vi "Check config.vi"(3 "error in (no error)":errorcluster, 4 "input cluster":T1 {"MaxLambdaCurrent [A]" format="%.2f"; "LambdaRates [A/min]" format="%.2f"; "MaxNormalCurrent [A]" format="%.2f"; "StabilitySetting [%]" format="%.2f"; "FieldCurrentRatio [T/A]" format="%.2f"; "SwitchWaitTime [s]" format="%.2f"; "SwitchHtrCurrent [mA]" format="%.2f"; "TrainRates [A/min]" format="%.2f"; "NormalRates [A/min]" format="%.2f"; "Breakpts [A]" format="%.2f"}, 5 "VISA session":refnum<visa-resource-name>="GPIB0::22::INSTR") -> (0 "error out":errorcluster, 1 "output cluster":T1 {"MaxLambdaCurrent [A]" format="%.2f"; "LambdaRates [A/min]" format="%.2f"; "MaxNormalCurrent [A]" format="%.2f"; "StabilitySetting [%]" format="%.2f"; "FieldCurrentRatio [T/A]" format="%.2f"; "SwitchWaitTime [s]" format="%.2f"; "SwitchHtrCurrent [mA]" format="%.2f"; "TrainRates [A/min]" format="%.2f"; "NormalRates [A/min]" format="%.2f"; "Breakpts [A]" format="%.2f"}, 2 "VISA session dup":refnum<visa-resource-name>)   [LabVIEW 2019]
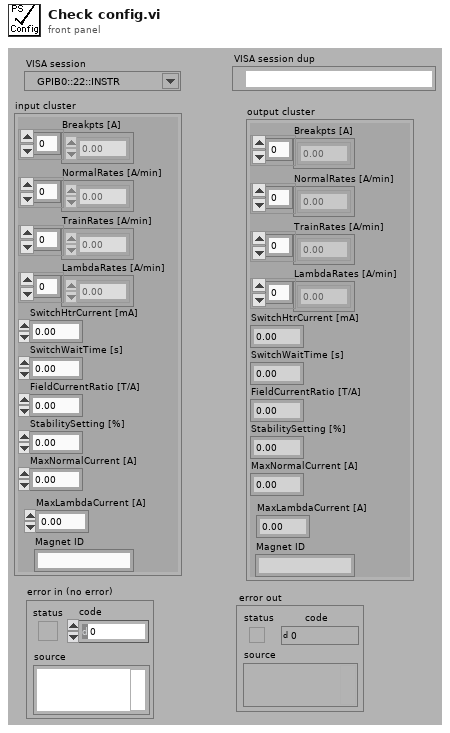
[diagram p1: front panel]
types:
  T1 = cluster{"Breakpts [A]":dbl[], "NormalRates [A/min]":dbl[], "TrainRates [A/min]":dbl[], "SwitchHtrCurrent [mA]":dbl, "SwitchWaitTime [s]":dbl, "FieldCurrentRatio [T/A]":dbl, "StabilitySetting [%]":dbl, "MaxNormalCurrent [A]":dbl, "Magnet ID":string, "LambdaRates [A/min]":dbl[], "MaxLambdaCurrent [A]":dbl}
  T2 = enum16{"SwitchHtrCurrent", "SwitchWaitTime", "FieldCurrentRatio", "StabilitySetting", "MaxNormalCurrent", "MaxLambdaCurrent"}
  T3 = enum16{"Normal", "Train", "Lambda", "Train & Lambda"}
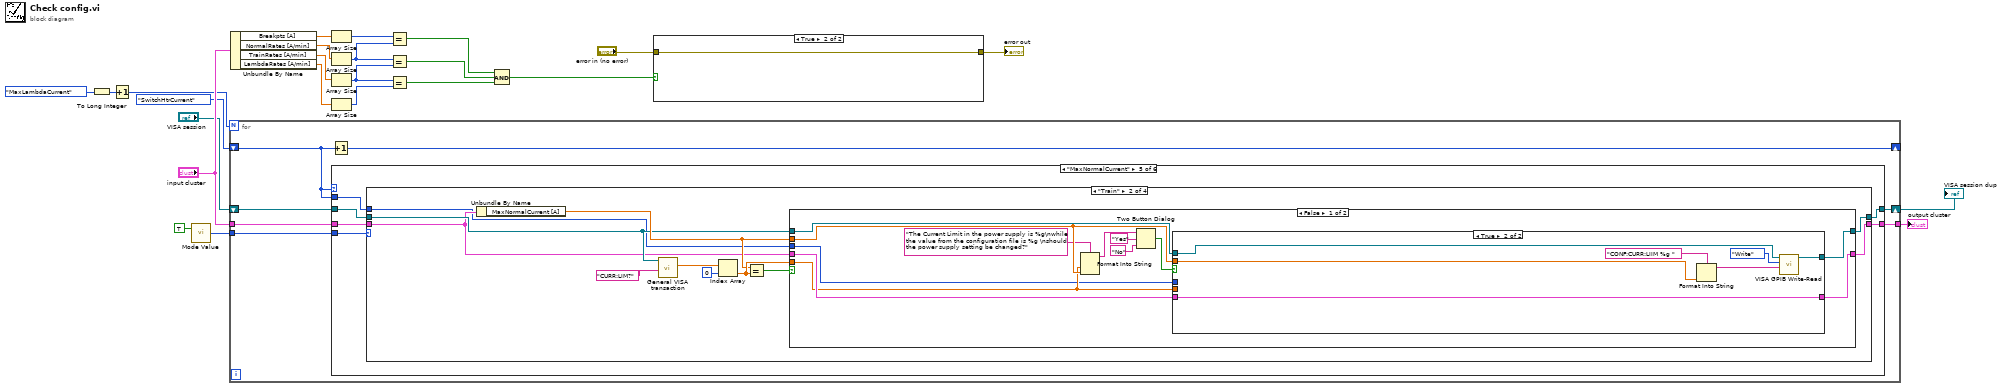
[diagram p0: block diagram]
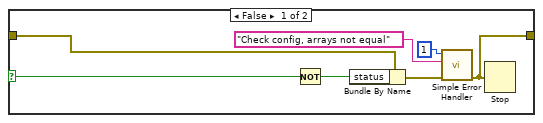
[diagram p2: hidden frame]
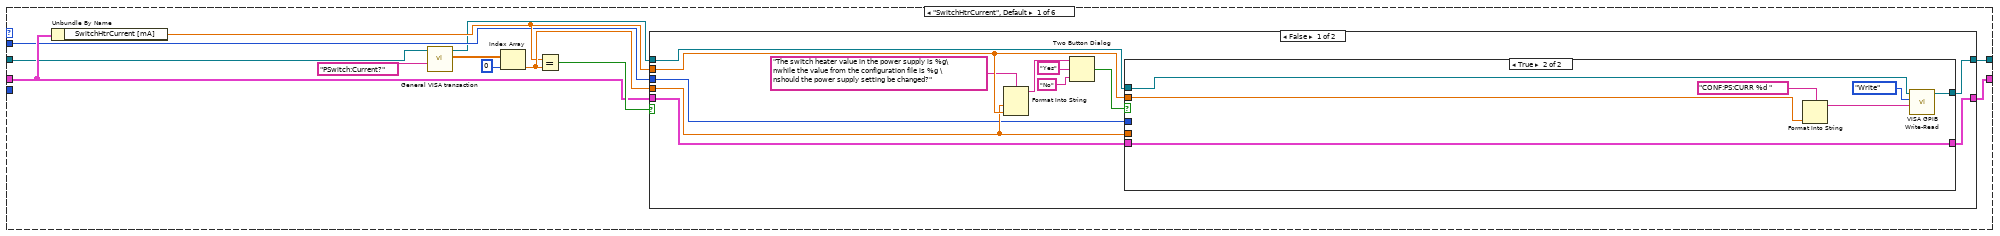
[diagram p3: hidden frame]
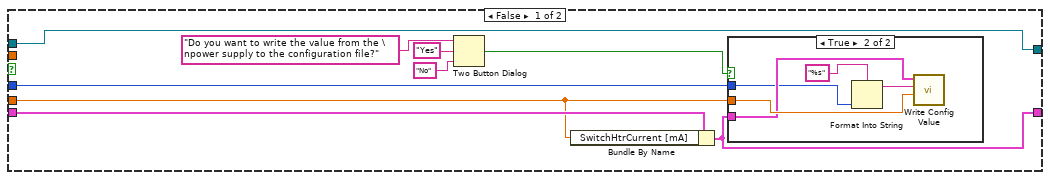
[diagram p4: hidden frame]
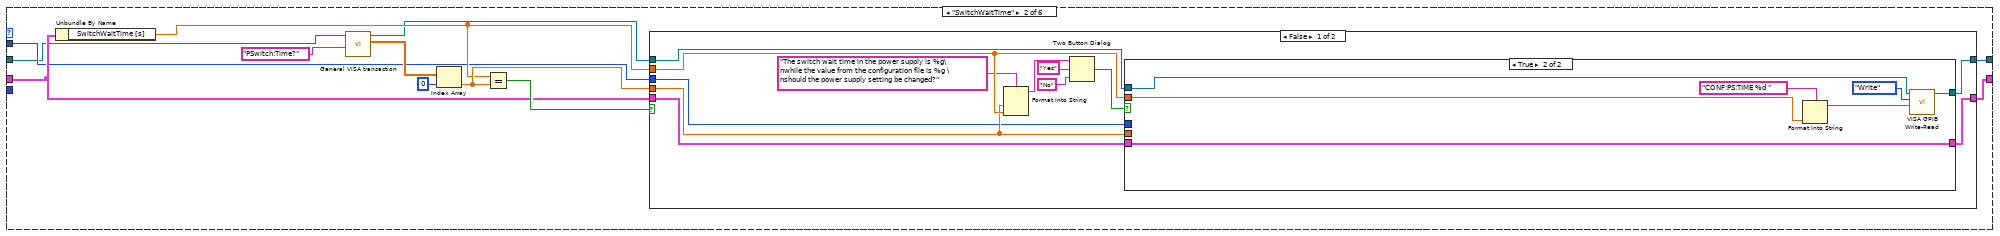
[diagram p7: hidden frame]
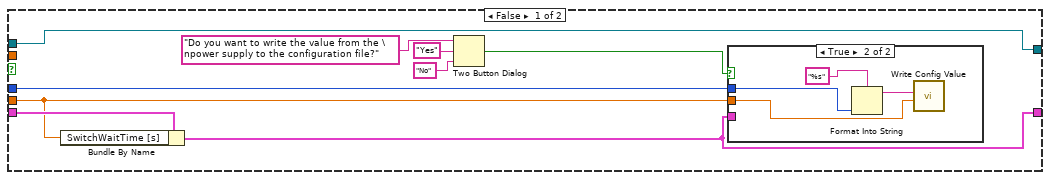
[diagram p8: hidden frame]
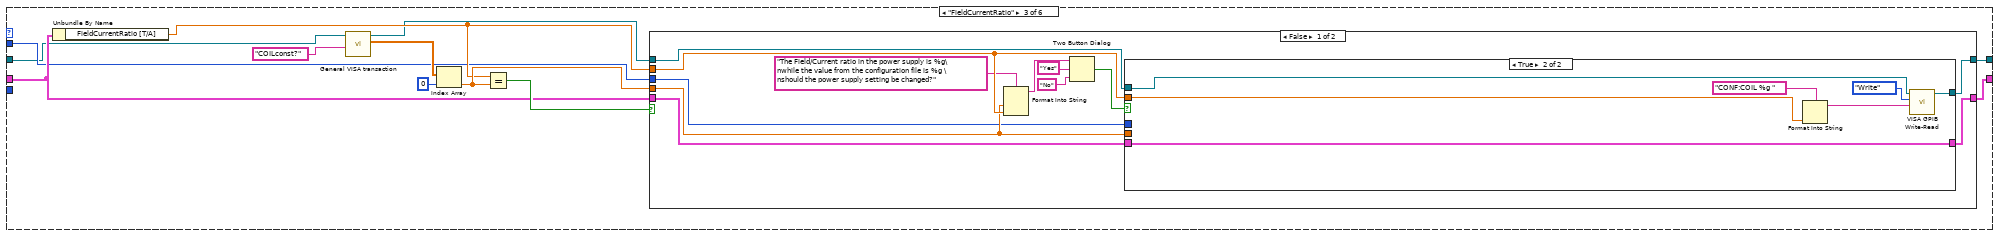
[diagram p11: hidden frame]
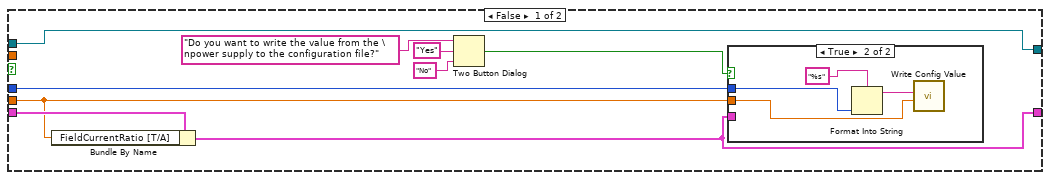
[diagram p12: hidden frame]
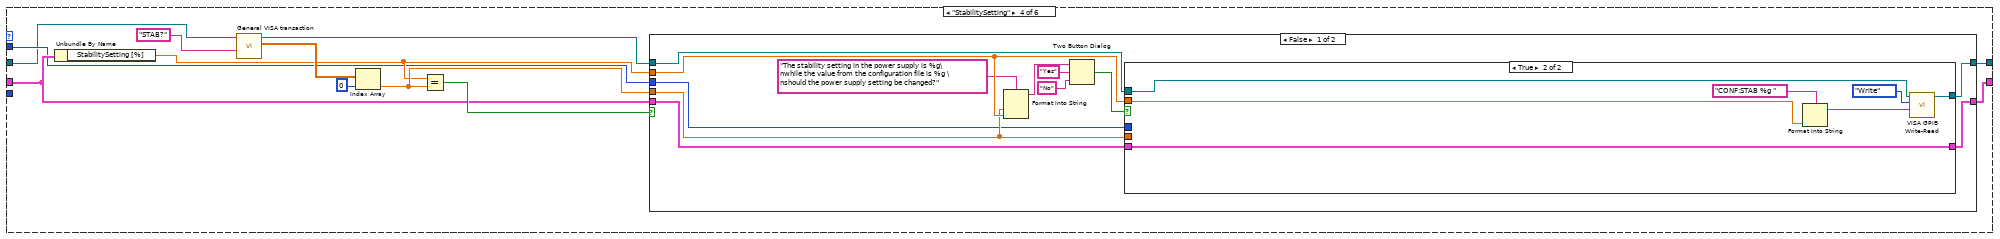
[diagram p15: hidden frame]
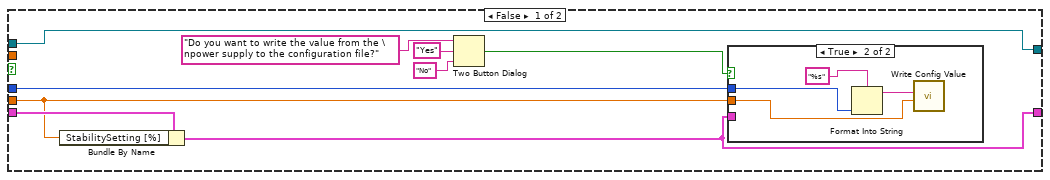
[diagram p16: hidden frame]
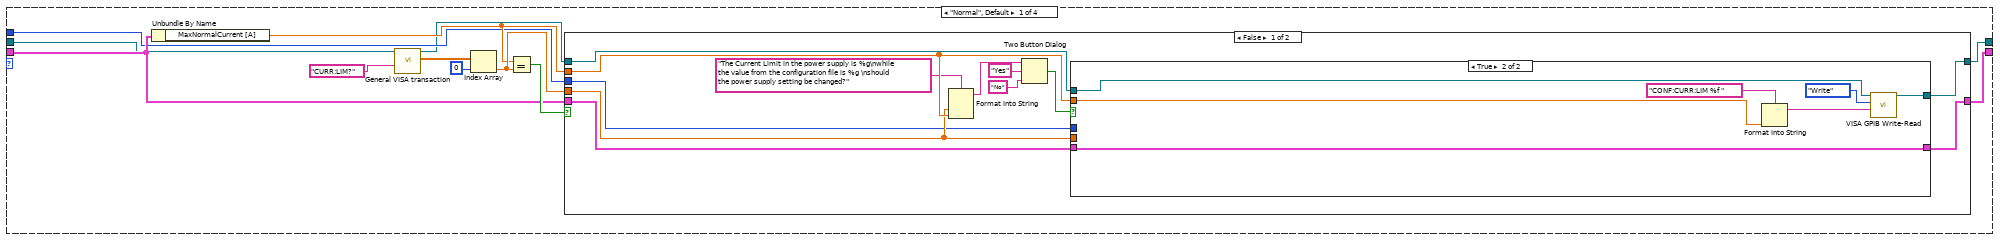
[diagram p19: hidden frame]
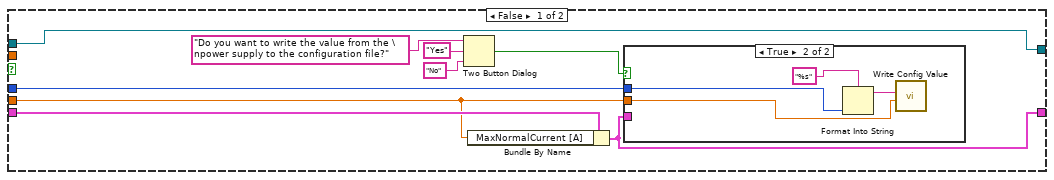
[diagram p20: hidden frame]
diagram:
  n1 = To Long Integer(number=T2."MaxLambdaCurrent") -> (32bit integer=w4:i32)
  n2 = Increment(x=w4) -> (x+1=w3:i32)
  n3 = call "Mode Value.vi"("Read/Write this vi"=TRUE) -> ("Mode Out"=w7:T3)  [unwired: 1 in]
  n4 = for {
    N: w3 -> [_]
    tunnel: "input cluster" -> [w31]
    tunnel: [w30] -> w6
    shift-right: [w29] -> _
    shift-left: T2."SwitchHtrCurrent" -> [w28]
    tunnel: w7 -> [w27]
    shift-right: [w25] -> w1
    shift-left: "VISA session" -> [w26]
    n5 = Increment(x=w28) -> (x+1=w29:T2)
    n6 = case shown="\"MaxNormalCurrent\"" w28 {
      tunnel: w26 -> [w34 w81 w126 w173 w222 w323]
      tunnel: w31 -> [w37 w84 w130 w176 w221 w322]
      tunnel: [w36 w83 w129 w175 w220 w321] -> w30
      tunnel: w28 -> [w35 w82 w128 w174 w219 w320]
      tunnel: w27 -> [_ _ _ _ w218 w319]
      tunnel: [w32 w79 w127 w171 w217 w318] -> w25
      frame "SwitchHtrCurrent", Default {
        n7 = Unbundle By Name(w37) -> ("SwitchHtrCurrent [mA]"=w38:dbl)
        n8 = call "General VISA transaction.vi"("Command String"="PSwitch:Current?", "VISA Session"=w34) -> ("Measurement"=w42:dbl[], "dup VISA Session"=w33:refnum<visa-resource-name>)  [unwired: 4 in, 4 out]
        n9 = Index Array(array=w42, index=0) -> (element=w39:dbl)
        n10 = Equal?(x=w38, y=w39) -> (x = y?=w40:bool)
        n11 = case shown="False" w40 {
          tunnel: w39 -> [w49 _]
          tunnel: w38 -> [w50 _]
          tunnel: w33 -> [w51 w77]
          tunnel: w37 -> [w47 w78]
          tunnel: [w46 w78] -> w36
          tunnel: w35 -> [w45 _]
          tunnel: [w44 w77] -> w32
          frame False {
            n12 = Format Into String(format string="The swItch heater value in the power supply is %g\nwhile the value from the configuration file is %g \nshould the power supply setting be changed?" ("message"), w49, w50) -> (resulting string=w55:string)  [unwired: 2 in, 1 out]
            n13 = Two Button Dialog(message=w55, 1:"No" ("F button name (\"Cancel\")"), 2:"Yes" ("T button name (\"OK\")")) -> (T button?=w52:bool)
            n14 = case shown="True" w52 {
              tunnel: w51 -> [w56 w75]
              tunnel: w50 -> [_ w74]
              tunnel: w49 -> [w59 _]
              tunnel: w47 -> [w60 w71]
              tunnel: [w58 w71] -> w46
              tunnel: w45 -> [w57 _]
              tunnel: [w56 w70] -> w44
              frame False {
                n15 = Two Button Dialog(message="Do you want to write the value from the \npower supply to the configuration file?", 1:"No" ("F button name (\"Cancel\")"), 2:"Yes" ("T button name (\"OK\")")) -> (T button?=w61:bool)
                n16 = Bundle By Name(cluster=w60, "SwitchHtrCurrent [mA]"=w59) -> (w58:T1)
                n17 = case shown="True" w61 {
                  tunnel: w59 -> [_ w69]
                  tunnel: w58 -> [_ w66]
                  tunnel: w57 -> [_ w65]
                  frame False {
                  }
                  frame True {
                    n18 = Format Into String(format string="%s", w65) -> (resulting string=w67:string)  [unwired: 2 in, 1 out]
                    n19 = call "Write Config Value.vi"("Value"=w69, "Key"=w67, "input cluster"=w66) -> ()  [unwired: 1 in, 2 out]
                  }
                }
              }
              frame True {
                n20 = Format Into String(format string="CONF:PS:CURR %d " ("Command String"), w74) -> (resulting string=w73:string)  [unwired: 2 in, 1 out]
                n21 = call "VISA GPIB Write-Read.vi"("Command"=w73, "Action"=enum16{"Write", "Read", "Write & Read"}."Write", "VISA resource name"=w75) -> ("dup VISA Session"=w70:refnum<visa-resource-name>)  [unwired: 5 in, 3 out]
              }
            }
          }
          frame True {
          }
        }
      }
      frame "SwitchWaitTime" {
        n22 = Unbundle By Name(w84) -> ("SwitchWaitTime [s]"=w85:dbl)
        n23 = call "General VISA transaction.vi"("Command String"="PSwitch:Time?", "VISA Session"=w81) -> ("Measurement"=w89:dbl[], "dup VISA Session"=w80:refnum<visa-resource-name>)  [unwired: 4 in, 4 out]
        n24 = Index Array(array=w89, index=0) -> (element=w86:dbl)
        n25 = Equal?(x=w85, y=w86) -> (x = y?=w87:bool)
        n26 = case shown="False" w87 {
          tunnel: w86 -> [w95 _]
          tunnel: w85 -> [w97 _]
          tunnel: w80 -> [w98 w123]
          tunnel: w84 -> [w94 w124]
          tunnel: [w93 w124] -> w83
          tunnel: w82 -> [w92 _]
          tunnel: [w91 w123] -> w79
          frame False {
            n27 = Format Into String(format string="The switch wait time in the power supply is %g\nwhile the value from the configuration file is %g \nshould the power supply setting be changed?" ("message"), w95, w97) -> (resulting string=w102:string)  [unwired: 2 in, 1 out]
            n28 = Two Button Dialog(message=w102, 1:"No" ("F button name (\"Cancel\")"), 2:"Yes" ("T button name (\"OK\")")) -> (T button?=w99:bool)
            n29 = case shown="True" w99 {
              tunnel: w98 -> [w103 w121]
              tunnel: w97 -> [_ w120]
              tunnel: w95 -> [w106 _]
              tunnel: w94 -> [w111 w117]
              tunnel: [w105 w117] -> w93
              tunnel: w92 -> [w104 _]
              tunnel: [w103 w116] -> w91
              frame False {
                n30 = Bundle By Name(cluster=w111, "SwitchWaitTime [s]"=w106) -> (w105:T1)
                n31 = Two Button Dialog(message="Do you want to write the value from the \npower supply to the configuration file?", 1:"No" ("F button name (\"Cancel\")"), 2:"Yes" ("T button name (\"OK\")")) -> (T button?=w107:bool)
                n32 = case shown="True" w107 {
                  tunnel: w106 -> [_ w115]
                  tunnel: w105 -> [_ _]
                  tunnel: w104 -> [_ w112]
                  frame False {
                  }
                  frame True {
                    n33 = Format Into String(format string="%s", w112) -> (resulting string=w113:string)  [unwired: 2 in, 1 out]
                    n34 = call "Write Config Value.vi"("Value"=w115, "Key"=w113) -> ()  [unwired: 2 in, 2 out]
                  }
                }
              }
              frame True {
                n35 = Format Into String(format string="CONF:PS:TIME %d " ("Command String"), w120) -> (resulting string=w119:string)  [unwired: 2 in, 1 out]
                n36 = call "VISA GPIB Write-Read.vi"("Command"=w119, "Action"=enum16{"Write", "Read", "Write & Read"}."Write", "VISA resource name"=w121) -> ("dup VISA Session"=w116:refnum<visa-resource-name>)  [unwired: 5 in, 3 out]
              }
            }
          }
          frame True {
          }
        }
      }
      frame "FieldCurrentRatio" {
        n37 = Unbundle By Name(w130) -> ("FieldCurrentRatio [T/A]"=w131:dbl)
        n38 = call "General VISA transaction.vi"("Command String"="COILconst?", "VISA Session"=w126) -> ("Measurement"=w135:dbl[], "dup VISA Session"=w125:refnum<visa-resource-name>)  [unwired: 4 in, 4 out]
        n39 = Index Array(array=w135, index=0) -> (element=w132:dbl)
        n40 = Equal?(x=w131, y=w132) -> (x = y?=w133:bool)
        n41 = case shown="False" w133 {
          tunnel: w132 -> [w139 _]
          tunnel: w131 -> [w143 _]
          tunnel: w125 -> [w144 w169]
          tunnel: w130 -> [w141 w170]
          tunnel: [w140 w170] -> w129
          tunnel: w128 -> [w138 _]
          tunnel: [w137 w169] -> w127
          frame False {
            n42 = Format Into String(format string="The Field/Current ratio in the power supply is %g\nwhile the value from the configuration file is %g \nshould the power supply setting be changed?" ("message"), w139, w143) -> (resulting string=w148:string)  [unwired: 2 in, 1 out]
            n43 = Two Button Dialog(message=w148, 1:"No" ("F button name (\"Cancel\")"), 2:"Yes" ("T button name (\"OK\")")) -> (T button?=w145:bool)
            n44 = case shown="True" w145 {
              tunnel: w144 -> [w149 w167]
              tunnel: w143 -> [_ w166]
              tunnel: w141 -> [w157 w163]
              tunnel: [w151 w163] -> w140
              tunnel: w139 -> [w152 _]
              tunnel: w138 -> [w150 _]
              tunnel: [w149 w162] -> w137
              frame False {
                n45 = Bundle By Name(cluster=w157, "FieldCurrentRatio [T/A]"=w152) -> (w151:T1)
                n46 = Two Button Dialog(message="Do you want to write the value from the \npower supply to the configuration file?", 1:"No" ("F button name (\"Cancel\")"), 2:"Yes" ("T button name (\"OK\")")) -> (T button?=w153:bool)
                n47 = case shown="True" w153 {
                  tunnel: w152 -> [_ w161]
                  tunnel: w151 -> [_ _]
                  tunnel: w150 -> [_ w158]
                  frame False {
                  }
                  frame True {
                    n48 = Format Into String(format string="%s", w158) -> (resulting string=w159:string)  [unwired: 2 in, 1 out]
                    n49 = call "Write Config Value.vi"("Value"=w161, "Key"=w159) -> ()  [unwired: 2 in, 2 out]
                  }
                }
              }
              frame True {
                n50 = Format Into String(format string="CONF:COIL %g " ("Command String"), w166) -> (resulting string=w165:string)  [unwired: 2 in, 1 out]
                n51 = call "VISA GPIB Write-Read.vi"("Command"=w165, "Action"=enum16{"Write", "Read", "Write & Read"}."Write", "VISA resource name"=w167) -> ("dup VISA Session"=w162:refnum<visa-resource-name>)  [unwired: 5 in, 3 out]
              }
            }
          }
          frame True {
          }
        }
      }
      frame "StabilitySetting" {
        n52 = Unbundle By Name(w176) -> ("StabilitySetting [%]"=w177:dbl)
        n53 = call "General VISA transaction.vi"("Command String"="STAB?", "VISA Session"=w173) -> ("Measurement"=w181:dbl[], "dup VISA Session"=w172:refnum<visa-resource-name>)  [unwired: 4 in, 4 out]
        n54 = Index Array(array=w181, index=0) -> (element=w178:dbl)
        n55 = Equal?(x=w177, y=w178) -> (x = y?=w179:bool)
        n56 = case shown="False" w179 {
          tunnel: w178 -> [w186 _]
          tunnel: w177 -> [w189 _]
          tunnel: w172 -> [w190 w215]
          tunnel: w176 -> [w187 w216]
          tunnel: [w185 w216] -> w175
          tunnel: w174 -> [w184 _]
          tunnel: [w183 w215] -> w171
          frame False {
            n57 = Format Into String(format string="The stability setting in the power supply is %g\nwhile the value from the configuration file is %g \nshould the power supply setting be changed?" ("message"), w186, w189) -> (resulting string=w194:string)  [unwired: 2 in, 1 out]
            n58 = Two Button Dialog(message=w194, 1:"No" ("F button name (\"Cancel\")"), 2:"Yes" ("T button name (\"OK\")")) -> (T button?=w191:bool)
            n59 = case shown="True" w191 {
              tunnel: w190 -> [w195 w213]
              tunnel: w189 -> [_ w212]
              tunnel: w187 -> [w203 w209]
              tunnel: w186 -> [w198 _]
              tunnel: [w197 w209] -> w185
              tunnel: w184 -> [w196 _]
              tunnel: [w195 w208] -> w183
              frame False {
                n60 = Bundle By Name(cluster=w203, "StabilitySetting [%]"=w198) -> (w197:T1)
                n61 = Two Button Dialog(message="Do you want to write the value from the \npower supply to the configuration file?", 1:"No" ("F button name (\"Cancel\")"), 2:"Yes" ("T button name (\"OK\")")) -> (T button?=w199:bool)
                n62 = case shown="True" w199 {
                  tunnel: w198 -> [_ w207]
                  tunnel: w197 -> [_ _]
                  tunnel: w196 -> [_ w204]
                  frame False {
                  }
                  frame True {
                    n63 = Format Into String(format string="%s", w204) -> (resulting string=w205:string)  [unwired: 2 in, 1 out]
                    n64 = call "Write Config Value.vi"("Value"=w207, "Key"=w205) -> ()  [unwired: 2 in, 2 out]
                  }
                }
              }
              frame True {
                n65 = Format Into String(format string="CONF:STAB %g " ("Command String"), w212) -> (resulting string=w211:string)  [unwired: 2 in, 1 out]
                n66 = call "VISA GPIB Write-Read.vi"("Command"=w211, "Action"=enum16{"Write", "Read", "Write & Read"}."Write", "VISA resource name"=w213) -> ("dup VISA Session"=w208:refnum<visa-resource-name>)  [unwired: 5 in, 3 out]
              }
            }
          }
          frame True {
          }
        }
      }
      frame "MaxNormalCurrent" {
        n67 = case shown="\"Train\"" w218 {
          tunnel: w222 -> [w225 w273 w314 w316]
          tunnel: w221 -> [w228 w272 w315 w317]
          tunnel: [w227 w271 w315 w317] -> w220
          tunnel: w219 -> [w226 w270 _ _]
          tunnel: [w223 w269 w314 w316] -> w217
          frame "Normal", Default {
            n68 = Unbundle By Name(w228) -> ("MaxNormalCurrent [A]"=w229:dbl)
            n69 = call "General VISA transaction.vi"("Command String"="CURR:LIM?", "VISA Session"=w225) -> ("Measurement"=w233:dbl[], "dup VISA Session"=w224:refnum<visa-resource-name>)  [unwired: 4 in, 4 out]
            n70 = Index Array(array=w233, index=0) -> (element=w230:dbl)
            n71 = Equal?(x=w229, y=w230) -> (x = y?=w231:bool)
            n72 = case shown="False" w231 {
              tunnel: w230 -> [w238 _]
              tunnel: w229 -> [w241 _]
              tunnel: w224 -> [w242 w267]
              tunnel: w228 -> [w239 w268]
              tunnel: [w237 w268] -> w227
              tunnel: w226 -> [w236 _]
              tunnel: [w235 w267] -> w223
              frame False {
                n73 = Format Into String(format string="The Current Limit in the power supply is %g\nwhile the value from the configuration file is %g \nshould the power supply setting be changed?" ("message"), w238, w241) -> (resulting string=w246:string)  [unwired: 2 in, 1 out]
                n74 = Two Button Dialog(message=w246, 1:"No" ("F button name (\"Cancel\")"), 2:"Yes" ("T button name (\"OK\")")) -> (T button?=w243:bool)
                n75 = case shown="True" w243 {
                  tunnel: w242 -> [w247 w265]
                  tunnel: w241 -> [_ w264]
                  tunnel: w239 -> [w255 w261]
                  tunnel: w238 -> [w250 _]
                  tunnel: [w249 w261] -> w237
                  tunnel: w236 -> [w248 _]
                  tunnel: [w247 w260] -> w235
                  frame False {
                    n76 = Two Button Dialog(message="Do you want to write the value from the \npower supply to the configuration file?", 1:"No" ("F button name (\"Cancel\")"), 2:"Yes" ("T button name (\"OK\")")) -> (T button?=w251:bool)
                    n77 = Bundle By Name(cluster=w255, "MaxNormalCurrent [A]"=w250) -> (w249:T1)
                    n78 = case shown="True" w251 {
                      tunnel: w250 -> [_ w259]
                      tunnel: w249 -> [_ _]
                      tunnel: w248 -> [_ w256]
                      frame False {
                      }
                      frame True {
                        n79 = Format Into String(format string="%s", w256) -> (resulting string=w257:string)  [unwired: 2 in, 1 out]
                        n80 = call "Write Config Value.vi"("Value"=w259, "Key"=w257) -> ()  [unwired: 2 in, 2 out]
                      }
                    }
                  }
                  frame True {
                    n81 = Format Into String(format string="CONF:CURR:LIM %f " ("Command String"), w264) -> (resulting string=w263:string)  [unwired: 2 in, 1 out]
                    n82 = call "VISA GPIB Write-Read.vi"("Command"=w263, "Action"=enum16{"Write", "Read", "Write & Read"}."Write", "VISA resource name"=w265) -> ("dup VISA Session"=w260:refnum<visa-resource-name>)  [unwired: 5 in, 3 out]
                  }
                }
              }
              frame True {
              }
            }
          }
          frame "Train" {
            n83 = Unbundle By Name(w272) -> ("MaxNormalCurrent [A]"=w274:dbl)
            n84 = call "General VISA transaction.vi"("Command String"="CURR:LIM?", "VISA Session"=w273) -> ("Measurement"=w278:dbl[])  [unwired: 4 in, 5 out]
            n85 = Index Array(array=w278, index=0) -> (element=w275:dbl)
            n86 = Equal?(x=w274, y=w275) -> (x = y?=w276:bool)
            n87 = case shown="False" w276 {
              tunnel: w275 -> [w283 _]
              tunnel: w274 -> [w286 _]
              tunnel: w273 -> [w287 w312]
              tunnel: w272 -> [w284 w313]
              tunnel: [w282 w313] -> w271
              tunnel: w270 -> [w281 _]
              tunnel: [w280 w312] -> w269
              frame False {
                n88 = Format Into String(format string="The Current Limit in the power supply is %g\nwhile the value from the configuration file is %g \nshould the power supply setting be changed?" ("message"), w283, w286) -> (resulting string=w291:string)  [unwired: 2 in, 1 out]
                n89 = Two Button Dialog(message=w291, 1:"No" ("F button name (\"Cancel\")"), 2:"Yes" ("T button name (\"OK\")")) -> (T button?=w288:bool)
                n90 = case shown="True" w288 {
                  tunnel: w287 -> [w292 w310]
                  tunnel: w286 -> [_ w309]
                  tunnel: w284 -> [w300 w306]
                  tunnel: w283 -> [w295 _]
                  tunnel: [w294 w306] -> w282
                  tunnel: w281 -> [w293 _]
                  tunnel: [w292 w305] -> w280
                  frame False {
                    n91 = Two Button Dialog(message="Do you want to write the value from the \npower supply to the configuration file?", 1:"No" ("F button name (\"Cancel\")"), 2:"Yes" ("T button name (\"OK\")")) -> (T button?=w296:bool)
                    n92 = Bundle By Name(cluster=w300, "MaxNormalCurrent [A]"=w295) -> (w294:T1)
                    n93 = case shown="True" w296 {
                      tunnel: w295 -> [_ w304]
                      tunnel: w294 -> [_ _]
                      tunnel: w293 -> [_ w301]
                      frame False {
                      }
                      frame True {
                        n94 = Format Into String(format string="%s", w301) -> (resulting string=w302:string)  [unwired: 2 in, 1 out]
                        n95 = call "Write Config Value.vi"("Value"=w304, "Key"=w302) -> ()  [unwired: 2 in, 2 out]
                      }
                    }
                  }
                  frame True {
                    n96 = Format Into String(format string="CONF:CURR:LIIM %g " ("Command String"), w309) -> (resulting string=w308:string)  [unwired: 2 in, 1 out]
                    n97 = call "VISA GPIB Write-Read.vi"("Command"=w308, "Action"=enum16{"Write", "Read", "Write & Read"}."Write", "VISA resource name"=w310) -> ("dup VISA Session"=w305:refnum<visa-resource-name>)  [unwired: 5 in, 3 out]
                  }
                }
              }
              frame True {
              }
            }
          }
          frame "Lambda" {
          }
          frame "Train & Lambda" {
          }
        }
      }
      frame "MaxLambdaCurrent" {
        n98 = case shown="\"Lambda\"" w319 {
          tunnel: w323 -> [w324 w326 w330 w375]
          tunnel: w322 -> [w325 w327 w333 w379]
          tunnel: [w325 w327 w332 w378] -> w321
          tunnel: w320 -> [_ _ w331 w377]
          tunnel: [w324 w326 w328 w376] -> w318
          frame "Normal", Default {
          }
          frame "Train" {
          }
          frame "Lambda" {
            n99 = Unbundle By Name(w333) -> ("MaxLambdaCurrent [A]"=w334:dbl)
            n100 = call "General VISA transaction.vi"("Command String"="CURR:LIM?", "VISA Session"=w330) -> ("Measurement"=w338:dbl[], "dup VISA Session"=w329:refnum<visa-resource-name>)  [unwired: 4 in, 4 out]
            n101 = Index Array(array=w338, index=0) -> (element=w335:dbl)
            n102 = Equal?(x=w334, y=w335) -> (x = y?=w336:bool)
            n103 = case shown="False" w336 {
              tunnel: w335 -> [w343 _]
              tunnel: w334 -> [w346 _]
              tunnel: w329 -> [w347 w372]
              tunnel: w333 -> [w344 w373]
              tunnel: [w342 w373] -> w332
              tunnel: w331 -> [w341 _]
              tunnel: [w340 w372] -> w328
              frame False {
                n104 = Format Into String(format string="The LambdaCurrent Limit in the power supply is %g\nwhile the value from the configuration file is %g \nshould the power supply setting be changed?" ("message"), w343, w346) -> (resulting string=w351:string)  [unwired: 2 in, 1 out]
                n105 = Two Button Dialog(message=w351, 1:"No" ("F button name (\"Cancel\")"), 2:"Yes" ("T button name (\"OK\")")) -> (T button?=w348:bool)
                n106 = case shown="True" w348 {
                  tunnel: w347 -> [w352 w370]
                  tunnel: w346 -> [_ w369]
                  tunnel: w344 -> [w360 w366]
                  tunnel: w343 -> [w355 _]
                  tunnel: [w354 w366] -> w342
                  tunnel: w341 -> [w353 _]
                  tunnel: [w352 w365] -> w340
                  frame False {
                    n107 = Two Button Dialog(message="Do you want to write the value from the \npower supply to the configuration file?", 1:"No" ("F button name (\"Cancel\")"), 2:"Yes" ("T button name (\"OK\")")) -> (T button?=w356:bool)
                    n108 = Bundle By Name(cluster=w360, "MaxNormalCurrent [A]"=w355) -> (w354:T1)
                    n109 = case shown="True" w356 {
                      tunnel: w355 -> [_ w364]
                      tunnel: w354 -> [_ _]
                      tunnel: w353 -> [_ w361]
                      frame False {
                      }
                      frame True {
                        n110 = Format Into String(format string="%s", w361) -> (resulting string=w362:string)  [unwired: 2 in, 1 out]
                        n111 = call "Write Config Value.vi"("Value"=w364, "Key"=w362) -> ()  [unwired: 2 in, 2 out]
                      }
                    }
                  }
                  frame True {
                    n112 = Format Into String(format string="CONF:CURR:LIM %g " ("Command String"), w369) -> (resulting string=w368:string)  [unwired: 2 in, 1 out]
                    n113 = call "VISA GPIB Write-Read.vi"("Command"=w368, "Action"=enum16{"Write", "Read", "Write & Read"}."Write", "VISA resource name"=w370) -> ("dup VISA Session"=w365:refnum<visa-resource-name>)  [unwired: 5 in, 3 out]
                  }
                }
              }
              frame True {
              }
            }
          }
          frame "Train & Lambda" {
            n114 = Unbundle By Name(w379) -> ("MaxNormalCurrent [A]"=w380:dbl)
            n115 = call "General VISA transaction.vi"("Command String"="CURR:LIM?", "VISA Session"=w375) -> ("Measurement"=w384:dbl[], "dup VISA Session"=w374:refnum<visa-resource-name>)  [unwired: 4 in, 4 out]
            n116 = Index Array(array=w384, index=0) -> (element=w381:dbl)
            n117 = Equal?(x=w380, y=w381) -> (x = y?=w382:bool)
            n118 = case shown="False" w382 {
              tunnel: w381 -> [w389 _]
              tunnel: w380 -> [w392 _]
              tunnel: w374 -> [w393 w418]
              tunnel: w379 -> [w390 w419]
              tunnel: [w388 w419] -> w378
              tunnel: w377 -> [w387 _]
              tunnel: [w386 w418] -> w376
              frame False {
                n119 = Format Into String(format string="The LambdaCurrent Limit in the power supply is %g\nwhile the value from the configuration file is %g \nshould the power supply setting be changed?" ("message"), w389, w392) -> (resulting string=w397:string)  [unwired: 2 in, 1 out]
                n120 = Two Button Dialog(message=w397, 1:"No" ("F button name (\"Cancel\")"), 2:"Yes" ("T button name (\"OK\")")) -> (T button?=w394:bool)
                n121 = case shown="True" w394 {
                  tunnel: w393 -> [w398 w416]
                  tunnel: w392 -> [_ w415]
                  tunnel: w390 -> [w406 w412]
                  tunnel: w389 -> [w401 _]
                  tunnel: [w400 w412] -> w388
                  tunnel: w387 -> [w399 _]
                  tunnel: [w398 w411] -> w386
                  frame False {
                    n122 = Two Button Dialog(message="Do you want to write the value from the \npower supply to the configuration file?", 1:"No" ("F button name (\"Cancel\")"), 2:"Yes" ("T button name (\"OK\")")) -> (T button?=w402:bool)
                    n123 = Bundle By Name(cluster=w406, "MaxNormalCurrent [A]"=w401) -> (w400:T1)
                    n124 = case shown="True" w402 {
                      tunnel: w401 -> [_ w410]
                      tunnel: w400 -> [_ _]
                      tunnel: w399 -> [_ w407]
                      frame False {
                      }
                      frame True {
                        n125 = Format Into String(format string="%s", w407) -> (resulting string=w408:string)  [unwired: 2 in, 1 out]
                        n126 = call "Write Config Value.vi"("Value"=w410, "Key"=w408) -> ()  [unwired: 2 in, 2 out]
                      }
                    }
                  }
                  frame True {
                    n127 = Format Into String(format string="CONF:CURR:LIIM %g " ("Command String"), w415) -> (resulting string=w414:string)  [unwired: 2 in, 1 out]
                    n128 = call "VISA GPIB Write-Read.vi"("Command"=w414, "Action"=enum16{"Write", "Read", "Write & Read"}."Write", "VISA resource name"=w416) -> ("dup VISA Session"=w411:refnum<visa-resource-name>)  [unwired: 5 in, 3 out]
                  }
                }
              }
              frame True {
              }
            }
          }
        }
      }
    }
  }
  "output cluster" <- w6
  "VISA session dup" <- w1
  n129 = Unbundle By Name("input cluster") -> ("Breakpts [A]"=w22:dbl[], "NormalRates [A/min]"=w24:dbl[], "TrainRates [A/min]"=w23:dbl[], "LambdaRates [A/min]"=w16:dbl[])
  n130 = Array Size(array=w22) -> (size(s)=w21:i32)
  n131 = Array Size(array=w24) -> (size(s)=w13:i32)
  n132 = Array Size(array=w23) -> (size(s)=w14:i32)
  n133 = Array Size(array=w16) -> (size(s)=w15:i32)
  n134 = Equal?(x=w21, y=w13) -> (x = y?=w12:bool)
  n135 = Equal?(x=w13, y=w14) -> (x = y?=w11:bool)
  n136 = Equal?(x=w14, y=w15) -> (x = y?=w10:bool)
  n137 = Compound Arithmetic op=AND(w12, w11, w10) -> (w19:bool)
  n138 = case shown="True" w19 {
    selector: w19 -> [w423 _]
    tunnel: "error in (no error)" -> [w426 w427]
    tunnel: [w421 w427] -> w18
    frame False {
      n139 = Not(x=w423) -> (.not. x?=w420:bool)
      n140 = Bundle By Name(cluster=w426, "status"=w420) -> (w425:errorcluster)
      n141 = call <vilib>:"Simple Error Handler.vi"("error code (no error:0)"=1, "error source (\" \")"="Check config, arrays not equal" ("error source (\" \")"), "error in (no error)"=w425) -> ("error out"=w421:errorcluster)  [unwired: 2 in, 4 out]
      n142 = Stop(stop? (T)=w421) -> ()
    }
    frame True {
    }
  }
  "error out" <- w18
